vi "LabJackT7.vi"(4 "Scan Period":dbl format="%.2f", 5 "Previous Scan Value":dbl format="%.2f", 6 "Present scan array":dbl[](array[numeric]) format="%.2f", 7 "Value to Output":dbl format="%.2f", 8 "Ch Description":T1={"Ch Name"="", "Type"="", "Function"=enum."Analogue Input", "Ch State"=enum."On", "Calibration type"=enum."Raw", "A"=0.0, "B"=0.0, "C"=0.0, "D"=0.0, "Comments"="", "Address"={"Main"=0, "Ch."=0, "Sub"=0, "Port Name"=""}, "String"="", "Duty"=65535} {"Duty" format="%.0b"; "D" format="%#_5g"; "C" format="%#_5g"; "B" format="%#_5g"; "A" format="%#_5g"}, 9 "Ch names":string[](array[string])) -> (0 "Scan comment":string, 1 "Output":dbl format="%.7f")   [LabVIEW 2013]
uses:
  ADAM Client/Sub VIs/ADAM Controls/Ch_description_ADAM.ctl
  ADAM Client/Sub VIs/ADAM Controls/Module_type_ADAM.ctl
  ADAM Client/Sub VIs/ADAM Controls/Function_ADAM.ctl
  ADAM Client/Sub VIs/ADAM Controls/Channel_State.ctl
  ADAM Client/Sub VIs/ADAM Controls/Calib_type_ADAM.ctl
  ADAM Client/Sub VIs/ADAM Controls/Address.ctl
  ADAM Client/Sub VIs/ADAM Controls/Remember_value_mode.ctl
  <vilib>/Utility/error.llb/DialogType.ctl
panel:
  in  "MaxAge(s)":dbl=1.5
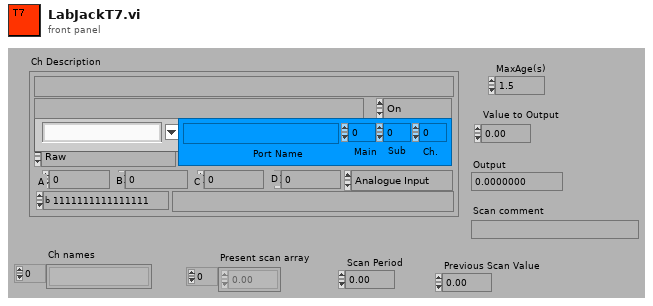
[diagram p1: front panel]
types:
  T1 = typedef "Ch_description_ADAM.ctl" = cluster{"Ch Name":string, "Type":T2, "Function":T3, "Ch State":T4, "Calibration type":T5, "A":dbl, "B":dbl, "C":dbl, "D":dbl, "Comments":string, "Address":T6, "String":string, "Duty":u16}
  T2 = typedef "Module_type_ADAM.ctl" = string
  T3 = typedef "Function_ADAM.ctl" = enum16{"Analogue Input", "Digital Input", "Event counter", "Event rate", "Analogue Output", "Digital Output", "Relay Output"}
  T4 = typedef "Channel_State.ctl" = enum16{"On", "Off", "Always On", "Always Off"}
  T5 = typedef "Calib_type_ADAM.ctl" = enum16{"Raw", "Bx + A", "Cx^2 + Bx + A", "Dx^3 + Cx^2 + Bx + A", "In Band", "Hi-Tec Q", "Hi-Tec M_dot", "Text"}
  T6 = typedef "Address.ctl" = cluster{"Main":i32, "Ch.":i32, "Sub":i32, "Port Name":string}
  T7 = typedef "Remember_value_mode.ctl" = enum16{"Read only", "Read and Write"}
  T8 = typedef "DialogType.ctl" = u16
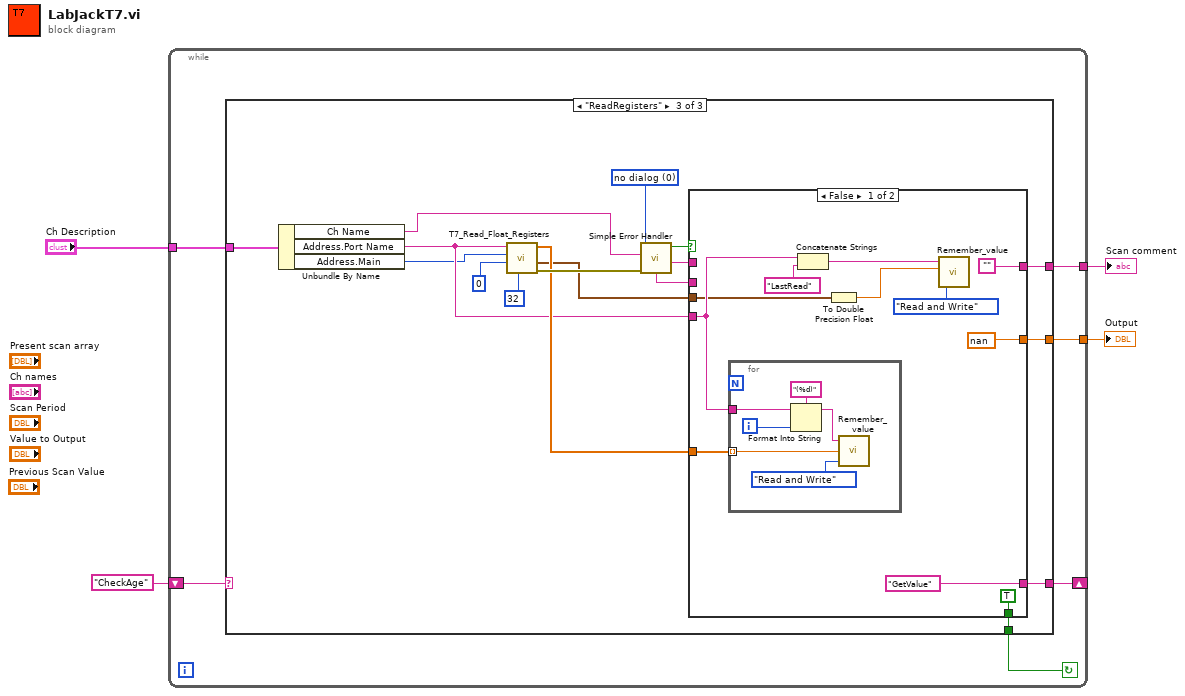
[diagram p0: block diagram]
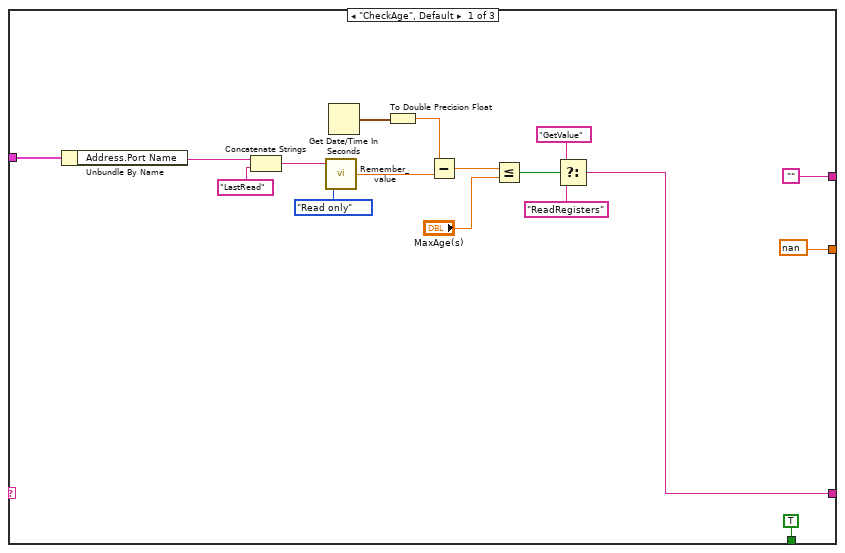
[diagram p2: hidden frame]
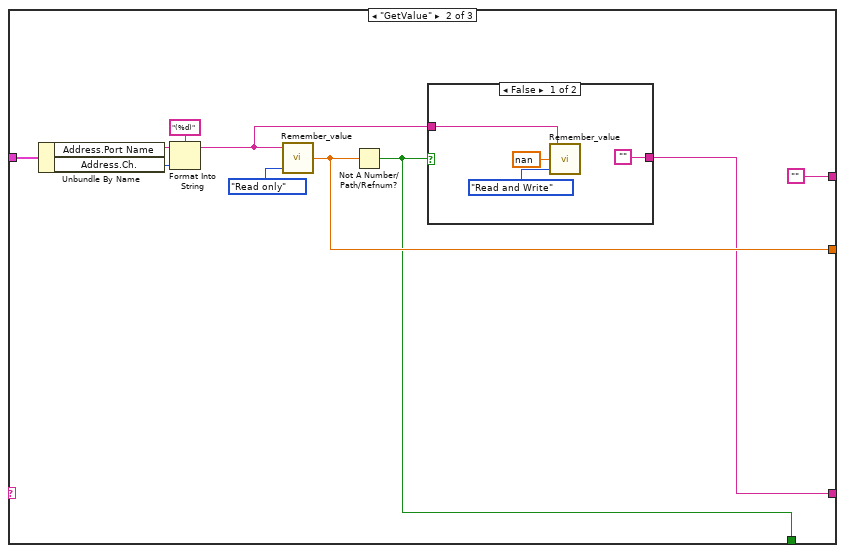
[diagram p3: hidden frame]
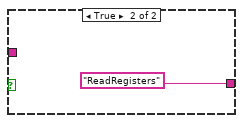
[diagram p4: hidden frame]
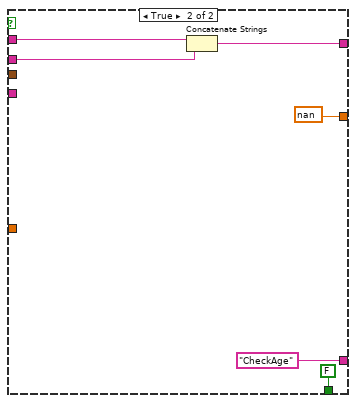
[diagram p5: hidden frame]
diagram:
  n1 = while {
    tunnel: "Ch Description" -> [w10]
    tunnel: [w9] -> w3
    shift-right: [w7] -> _
    shift-left: "CheckAge" -> [w8]
    tunnel: [w5] -> w1
    stop <- w6 continue-if-true
    n2 = case shown="\"ReadRegisters\"" w8 {
      tunnel: w10 -> [w24 w37 w59]
      tunnel: ["" "" w53] -> w9
      tunnel: [w14 w30 w47] -> w7
      tunnel: [TRUE w29 w44] -> w6
      tunnel: [nan w32 w43] -> w5
      frame "CheckAge", Default {
        n3 = Unbundle By Name(w24) -> ("Address.Port Name"=w23:string)
        n4 = Concatenate Strings(w23, "LastRead" ("string")) -> (w27:string)
        n5 = call "Remember_value.vi"("Mode"=Remember_value_mode."Read only", "Ch name"=w27) -> ("Output Value"=w20:dbl)  [unwired: 1 in]
        n6 = Get Date/Time In Seconds() -> (seconds since 1Jan1904=w22:timestamp)
        n7 = To Double Precision Float(number=w22) -> (double precision float=w21:dbl)
        n8 = Subtract(x=w21, y=w20) -> (x-y=w19:dbl)
        n9 = Less Or Equal?(x=w19, y="MaxAge(s)") -> (x <= y?=w17:bool)
        n10 = Select(t="GetValue", s=w17, f="ReadRegisters") -> (s? t:f=w14:string)
      }
      frame "GetValue" {
        n11 = Unbundle By Name(w37) -> ("Address.Port Name"=w33:string, "Address.Ch."=w34:i32)
        n12 = Format Into String(format string="(%d)", initial string=w33, w34) -> (resulting string=w28:string)  [unwired: 1 in, 1 out]
        n13 = call "Remember_value.vi"("Mode"=Remember_value_mode."Read only", "Ch name"=w28) -> ("Output Value"=w32:dbl)  [unwired: 1 in]
        n14 = Not A Number/Path/Refnum?(number/path/refnum=w32) -> (NaN/Path/Refnum?=w29:bool)
        n15 = case shown="False" w29 {
          tunnel: ["" "ReadRegisters"] -> w30
          tunnel: w28 -> [w40 _]
          frame False {
            n16 = call "Remember_value.vi"("Mode"=Remember_value_mode."Read and Write", "Input Value"=nan, "Ch name"=w40) -> ()  [unwired: 1 out]
          }
          frame True {
          }
        }
      }
      frame "ReadRegisters" {
        w58 = T8 0 items=["no dialog", "OK message", "continue or stop message", "OK message + warnings", "continue/stop + warnings"] ("type of dialog (OK msg:1)")
        n17 = Unbundle By Name(w59) -> ("Ch Name"=w55:string, "Address.Port Name"=w46:string, "Address.Main"=w45:i32)
        n18 = call "T7_Read_Float_Registers.vi"("Num Registers"=u16 32, "FirstChannel"=u16 0 ("Starting Address"), "Remote Port"=w45, "Remote IP Address"=w46) -> ("error out"=w52:errorcluster, "ReadAt"=w48:timestamp, "Array"=w49:dbl[])  [unwired: 4 in, 1 out]
        n19 = call <vilib>:"Simple Error Handler.vi"("error source (\" \")"=w55, "type of dialog (OK msg:1)"=w58, "error in (no error)"=w52) -> ("error?"=w54:bool, "source out"=w56:string, "message"=w57:string)  [unwired: 4 out]
        n20 = case shown="False" w54 {
          tunnel: w57 -> [_ w81]
          tunnel: w56 -> [_ w82]
          tunnel: ["" w80] -> w53
          tunnel: w46 -> [w66 _]
          tunnel: w49 -> [w65 _]
          tunnel: w48 -> [w64 _]
          tunnel: ["GetValue" "CheckAge"] -> w47
          tunnel: [TRUE FALSE] -> w44
          tunnel: [nan nan] -> w43
          frame False {
            n21 = for {
              tunnel: w65 -> [w76] mode=indexing
              tunnel: w66 -> [w75]
              i -> [w71]
              n22 = Format Into String(format string="(%d)", initial string=w75, w71) -> (resulting string=w74:string)  [unwired: 1 in, 1 out]
              n23 = call "Remember_value.vi"("Mode"=Remember_value_mode."Read and Write", "Input Value"=w76, "Ch name"=w74) -> ()  [unwired: 1 out]
            }
            n24 = Concatenate Strings(w66, "LastRead" ("string")) -> (w69:string)
            n25 = To Double Precision Float(number=w64) -> (double precision float=w63:dbl)
            n26 = call "Remember_value.vi"("Mode"=Remember_value_mode."Read and Write", "Input Value"=w63, "Ch name"=w69) -> ()  [unwired: 1 out]
          }
          frame True {
            n27 = Concatenate Strings(w82, w81) -> (w80:string)
          }
        }
      }
    }
  }
  "Output" <- w1
  "Scan comment" <- w3
